vi "gfitsio-insert-col.vi"(4 "tunits":string, 6 "tform":string, 7 "ttype":string, 8 "error in (no error)":errorcluster, 10 "insertion point (0:1st column)":i32, 11 "gfits refnum":T1) -> (0 "error out":errorcluster, 3 "dup gfits refnum":T1)   [LabVIEW 2011, in "gfitsio.lvlib"]
doc: "Insert a column in an ASCII or binary table. When inserting, <B>insertion point</B> specifies the column number that the new column should occupy in the table. Any existing columns from this position and higher are shifted over to allow room for the new column(s). The index number on all the following keywords will be incremented or decremented if necessary to reflect the new position of the column(s) in the table: TBCOLn, TFORMn, TTYPEn, TUNITn, TNULLn, TSCALn, TZEROn, TDISPn, TDIMn, TLMINn, TLMAXn, TDMINn, TDMAXn, TCTYPn, TCRPXn, TCRVLn, TCDLTn, TCROTn, and TCUNIn."
uses:
  gfitsio.lvlib
  gfitsio-refnum.ctl
  gfitsio.dll
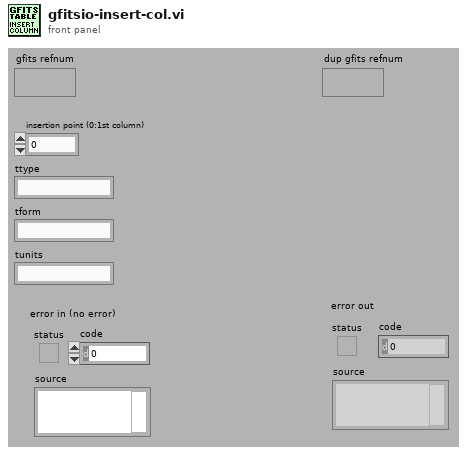
[diagram p1: front panel]
types:
  T1 = typedef "gfitsio.lvlib/gfitsio-refnum.ctl" = refnum<k1>
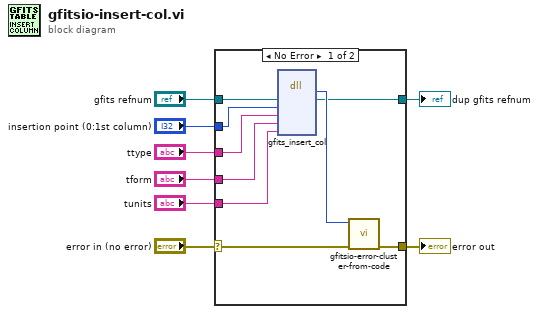
[diagram p0: block diagram]
diagram:
  n1 = case shown="No Error" "error in (no error)" {
    selector: "error in (no error)" -> [w15 w19]
    tunnel: [w17 w19] -> w1
    tunnel: "ttype" -> [w14 _]
    tunnel: "gfits refnum" -> [w12 w18]
    tunnel: [w13 w18] -> w2
    tunnel: "tform" -> [w11 _]
    tunnel: "insertion point (0:1st column)" -> [w10 _]
    tunnel: "tunits" -> [w9 _]
    frame No Error {
      n2 = dll-call lib="C:/BonOMM/BonOMM-SAOMM/SubVIs/gfitsio/gfitsio.dll" fn="gfits_insert_col"("gfits refnum"=w12, "colnum"=w10, "ttype"=w14, "tform"=w11, "tunits"=w9) -> (w16:i32, "gfits refnum"=w13:T1)  [unwired: 7 in, 2 out]
      n3 = call "gfitsio-error-cluster-from-code.vi"("error in (no error)"=w15, "error code"=w16) -> ("error out"=w17:errorcluster)  [unwired: 9 in]
    }
    frame Error {
    }
  }
  "error out" <- w1
  "dup gfits refnum" <- w2
